vi "Assert Equal_Float.vi"(4 "Use Percentage of X (F)":bool, 5 "Assert Only? (F)":bool, 6 "error code (1)":i32=1, 7 "Label":string, 8 "error in (no error)":errorcluster, 9 "Tolerance":ext=0.00000100000000000000000004, 10 "Y":ext, 11 "X":ext) -> (0 "error out":errorcluster)   [LabVIEW 2009, in "Caraya.lvlib" / "Assert.lvclass"]
doc: "Generates an error if the input condition is not met.\n\nTolerance is either an absolute or percentage value, depending on the \"Use Percentage of X\" flag. Defaults to absolute, tolerance = 1E-6.\nWhen Percentage mode, percentage is calculated based on value of X.\n\n\n--\nCopyright © 2015 JKI All rights reserved.\n\nAuthor: Tomi Maila <tomi.maila@jki.net>\n\nThis library is provided \"AS IS\" ,WITHOUT WARRANTIES OR\nCONDITIONS OF ANY KIND, either express or implied.\n\nJKI -- jki.net"
uses:
  Assert.lvclass
panel:
  # "Copyright © 2015 JKI All rights reserved.\n\nAuthor: Tomi Maila <tomi.maila@jki.net>\n\nThis library is provided \"AS IS\" ,WITHOUT WARRANTIES OR\nCONDITIONS OF ANY KIND, either express or implied.\n\nJKI -- jki.net"
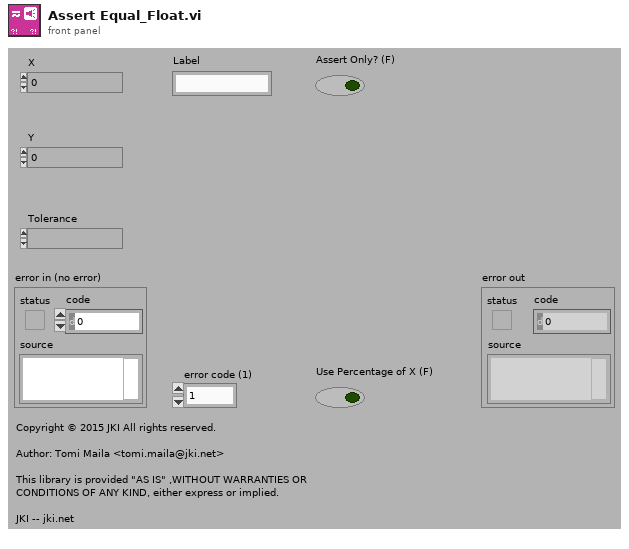
[diagram p1: front panel]
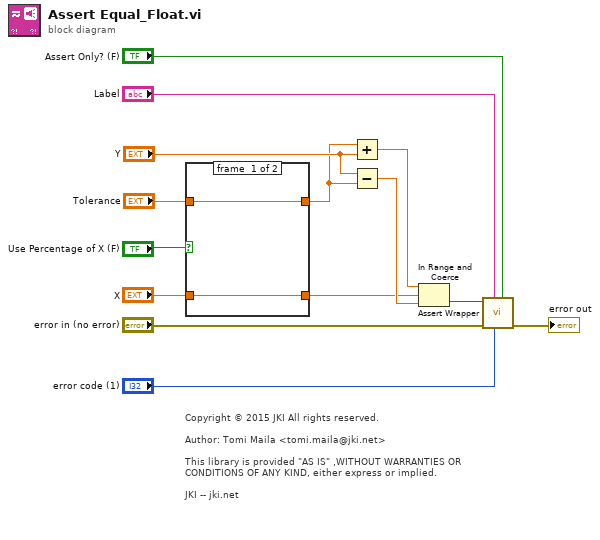
[diagram p0: block diagram]
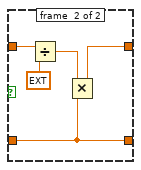
[diagram p2: hidden frame]
diagram:
  # "Copyright © 2015 JKI All rights reserved.\n\nAuthor: Tomi Maila <tomi.maila@jki.net>\n\nThis library is provided \"AS IS\" ,WITHOUT WARRANTIES OR\nCONDITIONS OF ANY KIND, either express or implied.\n\nJKI -- jki.net"
  n1 = case shown="True" "Use Percentage of X (F)" {
    tunnel: "Tolerance" -> [w16 w21]
    tunnel: [w16 w17] -> w3
    tunnel: "X" -> [w15 w18]
    tunnel: [w15 w18] -> w1
    frame #0 {
    }
    frame #1 {
      n2 = Divide(x=w21, y=ext 100.0) -> (x/y=w19:ext)
      n3 = Multiply(x=w19, y=w18) -> (x*y=w17:ext)
    }
  }
  n4 = Add(x=w3, y="Y") -> (x+y=w7:ext)
  n5 = Subtract(x="Y", y=w3) -> (x-y=w6:ext)
  n6 = In Range and Coerce(upper limit=w7, x=w1, lower limit=w6) -> (In Range?=w9:bool)  [unwired: 1 out]
  n7 = call "Assert Wrapper.vi"("Assert Only? (F)"="Assert Only? (F)", "error code (1)"="error code (1)", "Label"="Label", "error in (no error)"="error in (no error)", "Assert?"=w9) -> ("error out"=→"error out":errorcluster)  [unwired: 6 in]
